vi "2D Double Array to String.vi"(4 "Delimiter (,)":string=",", 6 "Numeric[][]":dbl[][](array[numeric])) -> (1 "String":string)   [LabVIEW 2016, in "SLL String.lvlib"]
uses:
  SLL String.lvlib
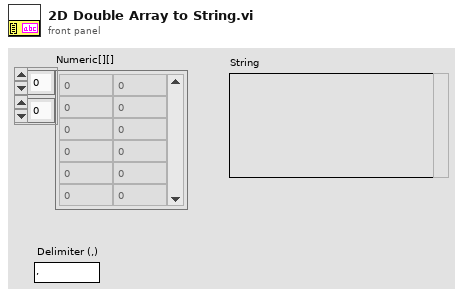
[diagram p1: front panel]
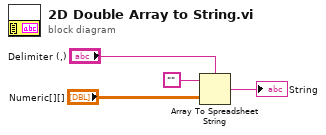
[diagram p0: block diagram]
diagram:
  n1 = Array To Spreadsheet String(delimiter (Tab)="Delimiter (,)", array="Numeric[][]", 3:"") -> (spreadsheet string=→"String":string)
